vi "HVAC Test.vi"(8 "error in":errorcluster, 11 "IED Test in":refnum<class "IED Test.lvclass">) -> (0 "error out":errorcluster, 2 "Test Result":T1=enum."Success", 3 "IED Test out":refnum<class "IED Test.lvclass">)   [LabVIEW 2018, in "IED Test Framework.lvlib" / "IED Test.lvclass"]
uses:
  IED Test.lvclass
  C:/Program Files (x86)/National Instruments/LabVIEW 2018/vi.lib/ActorFramework/Actor/Actor.lvclass
  C:/Users/Administrator/Desktop/2018LabVIEW EMS/EMS Generic Actor/EMS Generic/EMS Generic.lvclass
  Controls/Test Result.ctl
  <vilib>/ORNL/CSEISMIC DDS/CSEISMIC DDS Base/Data Types/Controls/DeviceClass Selector.ctl
  HVAC Actor/HVAC/HVAC.lvclass
  C:/Users/Administrator/Desktop/2018LabVIEW EMS/IED Actors/Device DDS Communications Framework/Device DDS Communications/Device DDS Communications.lvclass
  <vilib>/ORNL/CSEISMIC DDS/CSEISMIC DDS Base/CSEISMIC DDS.lvclass/CSEISMIC DDS.ctl
  <vilib>/ORNL/CSEISMIC DDS/CSEISMIC DDS Base/Data Types/Controls/DeviceID.ctl
  <vilib>/ActorFramework/Message Enqueuer/Message Enqueuer.lvclass/Message Enqueuer.ctl
  <vilib>/ORNL/CSEISMIC DDS/CSEISMIC DDS Base/Accessors/Write DDS Reference.vi
  <vilib>/ORNL/CSEISMIC DDS/CSEISMIC DDS Base/Accessors/Read DDS Reference.vi
  <vilib>/ActorFramework/Message Enqueuer/Enqueue.vi
  <vilib>/ORNL/CSEISMIC DDS/DDS Writer/DDS Writer.lvclass
  C:/Program Files (x86)/National Instruments/LabVIEW 2018/vi.lib/ORNL/CSEISMIC DDS/CSEISMIC DDS Base/CSEISMIC DDS.lvclass
  <vilib>/ActorFramework/Stop Msg/Stop Msg.lvclass
  C:/Program Files (x86)/National Instruments/LabVIEW 2018/vi.lib/ActorFramework/Message/Message.lvclass
  <vilib>/ORNL/CSEISMIC DDS/CSEISMIC DDS Base/Error Handler.vi
  <vilib>/ActorFramework/Message Priority Queue/Priority Enqueue.vi
  <vilib>/ORNL/CSEISMIC DDS/CSEISMIC DDS Base/CSEISMIC DDS.lvclass
  Device DDS Communications Framework/Device DDS Communications/Device DDS Communications.lvclass
  <vilib>/ActorFramework/Actor/Actor.lvclass
  EMS Generic Actor/EMS Generic/EMS Generic.lvclass
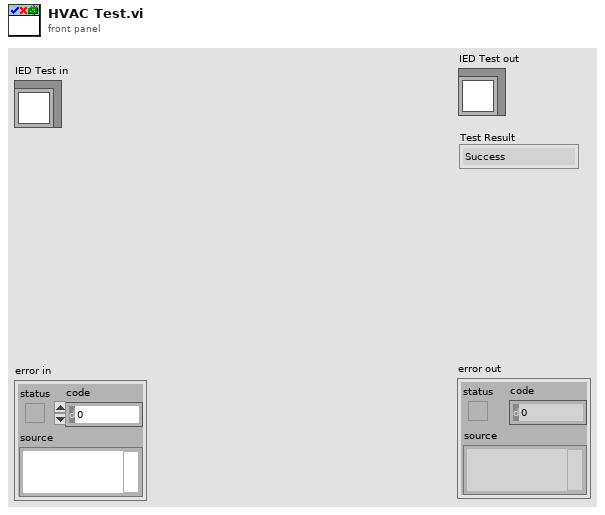
[diagram p1: front panel]
types:
  T1 = typedef "IED Test Framework.lvlib/IED Test.lvclass/Test Result.ctl" = enum16{"Invalid", "Success", "Failure", "Error", "Timeout"}
  T2 = typedef "CSEISMIC DDS.lvlib/CSEISMIC DDS.lvclass/DeviceID.ctl" = string
  T3 = typedef "CSEISMIC DDS.lvlib/CSEISMIC DDS.lvclass/DeviceClass Selector.ctl" = u16
  T4 = typedef "CSEISMIC DDS.lvlib/CSEISMIC DDS.lvclass/HVAC_Status.ctl" = cluster{"DeviceID":T2, "TemperatureSetpoint(degC)":dbl, "ControlMode":T5}
  T5 = typedef "CSEISMIC DDS.lvlib/CSEISMIC DDS.lvclass/ControlMode.ctl" = enum32{"Invalid", "Cooling", "Heating"}
  T6 = typedef "CSEISMIC DDS.lvlib/CSEISMIC DDS.lvclass/HVAC_Measurement.ctl" = cluster{"DeviceID":T2, "Temperature(degC)":dbl}
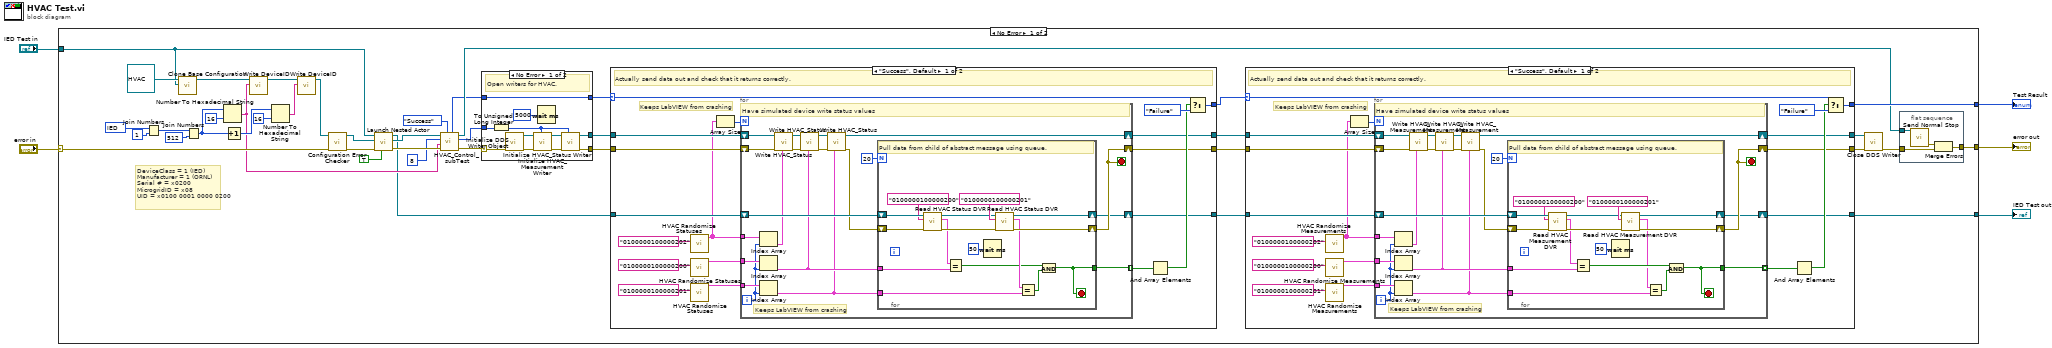
[diagram p0: block diagram]
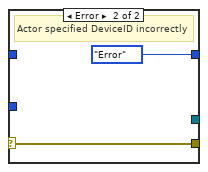
[diagram p4: hidden frame]
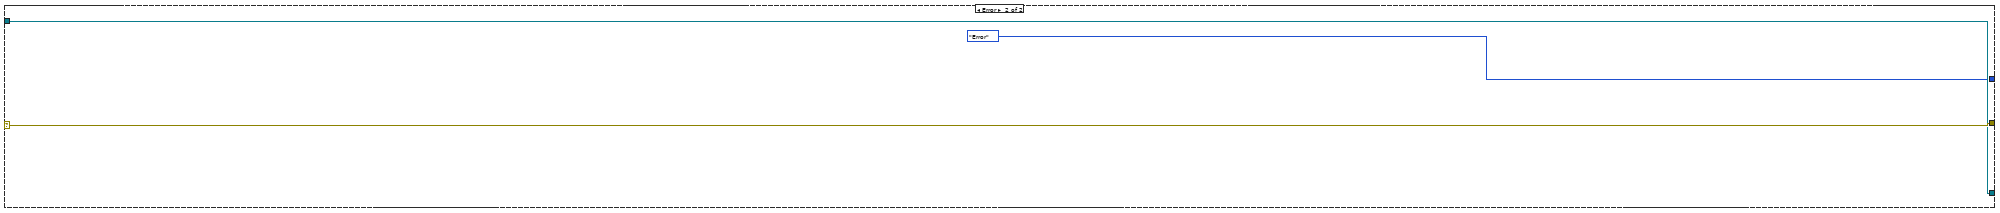
[diagram p5: hidden frame]
diagram:
  n1 = case shown="No Error" "error in" {
    selector: "error in" -> [w42 w182]
    tunnel: [w44 w182] -> w5
    tunnel: [w6 w181] -> w3
    tunnel: "IED Test in" -> [w9 w181]
    tunnel: [w22 Test_Result."Error" ("f")] -> w4
    frame No Error {
      w36 = T3 256 items=["Invalid"=0, "IED"=256, "DER"=512, "Relay"=768, "Meter"=1024, "Load"=1280, "Forecast"=1536, "Price"=1792, "Energy Storage"=513, "PV"=514, "Generator"=515, "Smart Relay"=769, "PCC"=770, "Smart Meter"=1025, "PMU"=1026, "HVAC"=1281] ("DeviceClass")
      # "DeviceClass = 1 (IED)\nManufacturer = 1 (ORNL)\nSerial # = x0200\nMicrogridID = x08\nUID = x0100 0001 0000 0200"
      n2 = Join Numbers(hi=w36, lo=u16 1 ("MicrogridID")) -> ((hi.lo)=w33:u32)
      n3 = call-dynamic "Clone Base Configuration.vi"("Source Object"=w9, "Target Object in"=refnum<class "HVAC.lvclass"> refnum ("HVAC Actor.lvlib:HVAC.lvclass")) -> ("Target Object out"=w10:refnum<class "HVAC.lvclass">)  [unwired: 9 in]
      n4 = Join Numbers(hi=w33, lo=u32 512 ("MicrogridID")) -> ((hi.lo)=w38:u64)
      n5 = Number To Hexadecimal String(1:i16 16 ("width (-)"), 2:w38) -> (0:w13:string)
      n6 = Increment(x=w38) -> (x+1=w40:u64)
      n7 = call-dynamic "Write DeviceID.vi"("DeviceID"=w13, "Device DDS Communications in"=w10) -> ("Device DDS Communications out"=w35:refnum<class "HVAC.lvclass">)  [unwired: 9 in]
      n8 = Number To Hexadecimal String(1:i16 16 ("width (-)"), 2:w40) -> (0:w41:string)
      n9 = call-dynamic "Write DeviceID.vi"("DeviceID"=w41, "Device DDS Communications in"=w35) -> ("Device DDS Communications out"=w21:refnum<class "HVAC.lvclass">)  [unwired: 9 in]
      n10 = call "Configuration Error Checker.vi"("error in"=w42, "Device DDS Communications in"=w21) -> ("error out"=w45:errorcluster, "Device DDS Communications out"=w43:refnum<class "HVAC.lvclass">)  [unwired: 8 in]
      n11 = call <vilib>:"Launch Nested Actor.vi"("Open Actor Core front panel? (F)"=TRUE, "error in (no error)"=w45, "Nested Actor"=w43, "Caller Actor in"=w9) -> ("error out"=w19:errorcluster, "Nested Actor's Enqueuer"=w15:refnum<class "Message Enqueuer.lvclass">, "Caller Actor out"=w7:refnum<class "IED Test.lvclass">)  [unwired: 5 in]
      n12 = call "HVAC_Control_subTest.vi"("Test Result in"=Test_Result."Success", "error in"=w19, "DeviceID"=w13, "MicrogridID"=u8 8 ("domain id"), "Message Enqueuer in"=w15) -> ("error out"=w18:errorcluster, "dup MicrogridID"=w16:u8, "Message Enqueuer out"=w14:refnum<class "Message Enqueuer.lvclass">, "Test Result out"=w12:T1)  [unwired: 2 in, 1 out]
      n13 = case shown="No Error" w18 {
        selector: w18 -> [w175 w179]
        tunnel: [w169 w179] -> w29
        tunnel: w16 -> [w177 _]
        tunnel: [w167 Test_Result."Error" ("Test Result")] -> w31
        tunnel: [w168 _] -> w30
        tunnel: w12 -> [w167 _]
        frame No Error {
          # "Open writers for HVAC."
          n14 = To Unsigned Long Integer(number=w177) -> (unsigned 32bit integer=w170:u32)
          n15 = call <vilib>:"Initialize DDS Writer Object.vi"("error in"=w175) -> ("error out"=w174:errorcluster, "DDS Writer out"=w173:refnum<class "DDS Writer.lvclass">)  [unwired: 9 in]
          n16 = call <vilib>:"Initialize HVAC_Measurement Writer.vi"("MicrogridID"=w170, "error in"=w174, "DDS Writer in"=w173) -> ("error out"=w171:errorcluster, "DDS Writer"=w172:refnum<class "DDS Writer.lvclass">)  [unwired: 7 in]
          n17 = Wait (ms)(milliseconds to wait=u32 5000) -> ()  [unwired: 1 out]
          n18 = call <vilib>:"Initialize HVAC_Status Writer.vi"("MicrogridID"=w170, "error in"=w171, "DDS Writer in"=w172) -> ("error out"=w169:errorcluster, "DDS Writer out"=w168:refnum<class "DDS Writer.lvclass">)  [unwired: 7 in]
        }
        frame Error {
          # "Actor specified DeviceID incorrectly"
        }
      }
      n19 = case shown="\"Success\", Default" w31 {
        selector: w31 -> [w67 w107]
        tunnel: w30 -> [w68 w106]
        tunnel: w7 -> [w62 w105]
        tunnel: w29 -> [w63 w108]
        tunnel: [w65 w107] -> w26
        tunnel: [w61 w108] -> w27
        tunnel: [w59 w106] -> w28
        tunnel: [w52 w105] -> w8
        frame "Success", Default {
          # "Keeps LabVIEW from crashing"
          # "Actually send data out and check that it returns correctly."
          n20 = call "HVAC Randomize Statuses.vi"("DeviceID"=T2 "0100000100000202" ("(hi.lo)")) -> ("HVAC_Status Array out"=w58:T4[])  [unwired: 10 in]
          n21 = call "HVAC Randomize Statuses.vi"("DeviceID"=T2 "0100000100000200" ("(hi.lo)")) -> ("HVAC_Status Array out"=w53:T4[])  [unwired: 10 in]
          n22 = call "HVAC Randomize Statuses.vi"("DeviceID"=T2 "0100000100000201" ("(hi.lo)")) -> ("HVAC_Status Array out"=w54:T4[])  [unwired: 10 in]
          n23 = Array Size(array=w58) -> (size(s)=w60:i32)
          n24 = for {
            N: w60 -> [_]
            shift-right: [w85] -> w59
            shift-left: w68 -> [w88]
            tunnel: w58 -> [w81]
            tunnel: w54 -> [w76]
            tunnel: w53 -> [w77]
            shift-right: [w78] -> w61
            shift-left: w63 -> [w84]
            shift-right: [w72] -> w52
            shift-left: w62 -> [w80]
            tunnel: [w69] -> w51 mode=indexing
            i -> [w74]
            stop <- w78 stop-if-true
            # "Keeps LabVIEW from crashing"
            # "Have simulated device write status values"
            n25 = Index Array(array=w81, index=w74) -> (element=w73:T4)
            n26 = Index Array(array=w77, index=w74) -> (element=w71:T4)
            n27 = Index Array(array=w76, index=w74) -> (element=w70:T4)
            n28 = call <vilib>:"Write HVAC_Status.vi"("HVAC_Status"=w73, "error in"=w84, "DDS Writer in"=w88) -> ("error out"=w83:errorcluster, "DDS Writer out"=w87:refnum<class "DDS Writer.lvclass">)  [unwired: 7 in]
            n29 = call <vilib>:"Write HVAC_Status.vi"("HVAC_Status"=w71, "error in"=w83, "DDS Writer in"=w87) -> ("error out"=w82:errorcluster, "DDS Writer out"=w86:refnum<class "DDS Writer.lvclass">)  [unwired: 7 in]
            n30 = call <vilib>:"Write HVAC_Status.vi"("HVAC_Status"=w70, "error in"=w82, "DDS Writer in"=w86) -> ("error out"=w79:errorcluster, "DDS Writer out"=w85:refnum<class "DDS Writer.lvclass">)  [unwired: 7 in]
            n31 = for {
              N: 20 -> [_]
              shift-right: [w97] -> w78
              shift-left: w79 -> [w103]
              shift-right: [w98] -> w72
              shift-left: w80 -> [w104]
              tunnel: w71 -> [w95]
              tunnel: w70 -> [w93]
              tunnel: [w90] -> w69
              stop <- w90 stop-if-true
              # "Pull data from child of abstract message using queue."
              n32 = call "Read HVAC Status DVR.vi"("error in"=w103, "DeviceID"=T2 "0100000100000200" ("(hi.lo)"), "EMS Generic in"=w104) -> ("error out"=w100:errorcluster, "HVAC_Status"=w96:T4, "EMS Generic out"=w99:refnum<class "IED Test.lvclass">)  [unwired: 5 in, 1 out]
              n33 = Equal?(x=w96, y=w95) -> (x = y?=w92:bool)
              n34 = Wait (ms)(milliseconds to wait=u32 50) -> ()  [unwired: 1 out]
              n35 = call "Read HVAC Status DVR.vi"("error in"=w100, "DeviceID"=T2 "0100000100000201" ("(hi.lo)"), "EMS Generic in"=w99) -> ("error out"=w97:errorcluster, "HVAC_Status"=w94:T4, "EMS Generic out"=w98:refnum<class "IED Test.lvclass">)  [unwired: 5 in, 1 out]
              n36 = Equal?(x=w94, y=w93) -> (x = y?=w91:bool)
              n37 = And(x=w92, y=w91) -> (x .and. y?=w90:bool)
            }
          }
          n38 = And Array Elements(Boolean array=w51) -> (logical AND=w64:bool)
          n39 = Select(t=w67, s=w64, f=Test_Result."Failure") -> (s? t:f=w65:T1)
        }
        frame "Error" {
        }
      }
      n40 = case shown="\"Success\", Default" w26 {
        selector: w26 -> [w125 w165]
        tunnel: w28 -> [w126 w164]
        tunnel: w8 -> [w120 w163]
        tunnel: w27 -> [w121 w166]
        tunnel: [w123 w165] -> w22
        tunnel: [w119 w166] -> w24
        tunnel: [w117 w164] -> w25
        tunnel: [w109 w163] -> w6
        frame "Success", Default {
          # "Keeps LabVIEW from crashing"
          # "Actually send data out and check that it returns correctly."
          n41 = call "HVAC Randomize Measurements.vi"("DeviceID"=T2 "0100000100000202" ("(hi.lo)")) -> ("HVAC_Measurement Array out"=w116:T6[])  [unwired: 10 in]
          n42 = call "HVAC Randomize Measurements.vi"("DeviceID"=T2 "0100000100000200" ("(hi.lo)")) -> ("HVAC_Measurement Array out"=w111:T6[])  [unwired: 10 in]
          n43 = call "HVAC Randomize Measurements.vi"("DeviceID"=T2 "0100000100000201" ("(hi.lo)")) -> ("HVAC_Measurement Array out"=w112:T6[])  [unwired: 10 in]
          n44 = Array Size(array=w116) -> (size(s)=w118:i32)
          n45 = for {
            N: w118 -> [_]
            shift-right: [w143] -> w117
            shift-left: w126 -> [w146]
            tunnel: w116 -> [w139]
            tunnel: w112 -> [w134]
            tunnel: w111 -> [w135]
            shift-right: [w136] -> w119
            shift-left: w121 -> [w142]
            shift-right: [w130] -> w109
            shift-left: w120 -> [w138]
            tunnel: [w127] -> w110 mode=indexing
            i -> [w132]
            stop <- w136 stop-if-true
            # "Keeps LabVIEW from crashing"
            # "Have simulated device write status values"
            n46 = Index Array(array=w139, index=w132) -> (element=w131:T6)
            n47 = Index Array(array=w135, index=w132) -> (element=w129:T6)
            n48 = Index Array(array=w134, index=w132) -> (element=w128:T6)
            n49 = call <vilib>:"Write HVAC_Measurement.vi"("HVAC_Measurement"=w131, "error in"=w142, "DDS Writer in"=w146) -> ("error out"=w141:errorcluster, "DDS Writer out"=w145:refnum<class "DDS Writer.lvclass">)  [unwired: 7 in]
            n50 = call <vilib>:"Write HVAC_Measurement.vi"("HVAC_Measurement"=w129, "error in"=w141, "DDS Writer in"=w145) -> ("error out"=w140:errorcluster, "DDS Writer out"=w144:refnum<class "DDS Writer.lvclass">)  [unwired: 7 in]
            n51 = call <vilib>:"Write HVAC_Measurement.vi"("HVAC_Measurement"=w128, "error in"=w140, "DDS Writer in"=w144) -> ("error out"=w137:errorcluster, "DDS Writer out"=w143:refnum<class "DDS Writer.lvclass">)  [unwired: 7 in]
            n52 = for {
              N: 20 -> [_]
              shift-right: [w152] -> w136
              shift-left: w137 -> [w161]
              shift-right: [w153] -> w130
              shift-left: w138 -> [w162]
              tunnel: w129 -> [w149]
              tunnel: w128 -> [w148]
              tunnel: [w147] -> w127
              stop <- w147 stop-if-true
              # "Pull data from child of abstract message using queue."
              n53 = call "Read HVAC Measurement DVR.vi"("error in"=w161, "DeviceID"=T2 "0100000100000200" ("(hi.lo)"), "EMS Generic in"=w162) -> ("error out"=w157:errorcluster, "HVAC_Measurement"=w150:T6, "EMS Generic out"=w158:refnum<class "IED Test.lvclass">)  [unwired: 5 in, 1 out]
              n54 = Equal?(x=w150, y=w149) -> (x = y?=w154:bool)
              n55 = Wait (ms)(milliseconds to wait=u32 50) -> ()  [unwired: 1 out]
              n56 = call "Read HVAC Measurement DVR.vi"("error in"=w157, "DeviceID"=T2 "0100000100000201" ("(hi.lo)"), "EMS Generic in"=w158) -> ("error out"=w152:errorcluster, "HVAC_Measurement"=w151:T6, "EMS Generic out"=w153:refnum<class "IED Test.lvclass">)  [unwired: 5 in, 1 out]
              n57 = Equal?(x=w151, y=w148) -> (x = y?=w155:bool)
              n58 = And(x=w154, y=w155) -> (x .and. y?=w147:bool)
            }
          }
          n59 = And Array Elements(Boolean array=w110) -> (logical AND=w122:bool)
          n60 = Select(t=w125, s=w122, f=Test_Result."Failure") -> (s? t:f=w123:T1)
        }
        frame "Error" {
        }
      }
      n61 = call <vilib>:"Close DDS Writer.vi"("error in"=w24, "DDS Writer in"=w25) -> ("error out"=w23:errorcluster)  [unwired: 9 in]
      n62 = flat-sequence {
        tunnel: w14 -> [w50]
        tunnel: [w48] -> w44
        tunnel: w23 -> [w47]
        frame #0 {
          n63 = call <vilib>:"Send Normal Stop.vi"("Message Enqueuer"=w50) -> ("error out"=w49:errorcluster)  [unwired: 10 in]
          n64 = Merge Errors(w49, w47) -> (w48:errorcluster)
        }
      }
    }
    frame Error {
    }
  }
  "error out" <- w5
  "IED Test out" <- w3
  "Test Result" <- w4
